vi "Set Cursor.vi"   [LabVIEW 2020]
doc: "Changes the appearance of the cursor on the front panel of a VI. Wire data to the <B>icon</B> input to determine the polymorphic instance to use or manually select the instance."
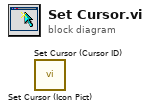
[diagram p0: block diagram]
diagram:
  n1 = call "Set Cursor (Icon Pict).vi"() -> ()  [unwired: 10 in, 2 out]
  n2 = call "Set Cursor (Cursor ID).vi"() -> ()  [unwired: 10 in, 2 out]
